vi "API_GetWindowhWnd by Window Name.vi"(8 "error in (no error)":errorcluster caption="错误输入（无错误）", 11 "窗口名称 (\"\")":string) -> (0 "error out":errorcluster caption="错误输出", 3 "窗口句柄(0)":i32)   [LabVIEW 2012, in "API.lvlib"]
uses:
  API.lvlib
  user32.dll
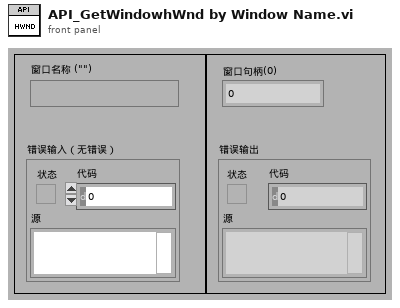
[diagram p1: front panel]
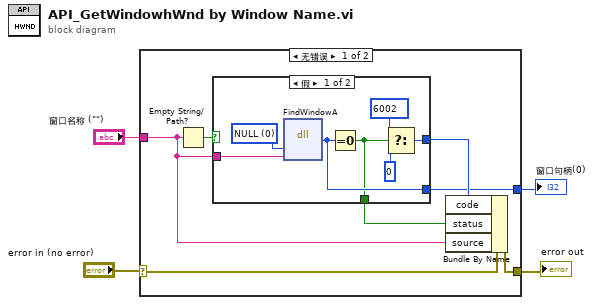
[diagram p0: block diagram]
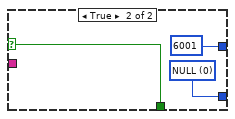
[diagram p2: hidden frame]
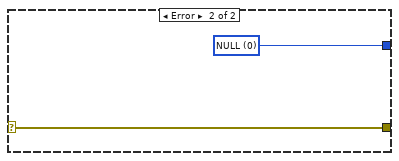
[diagram p3: hidden frame]
diagram:
  n1 = case shown="无错误" "error in (no error)" {
    selector: "error in (no error)" -> [w6 w22]
    tunnel: [w9 w22] -> w1
    tunnel: [w8 w23] -> w4
    tunnel: "窗口名称 (\"\")" -> [w5 _]
    frame No Error {
      n2 = Empty String/Path?(string/path=w5) -> (empty?=w7:bool)
      n3 = case shown="假" w7 {
        selector: w7 -> [_ w19]
        tunnel: [w18 w20] -> w8
        tunnel: [w17 w19] -> w10
        tunnel: [w16 6001] -> w11
        tunnel: w5 -> [w12 _]
        frame False {
          w13 = 0 items=["NULL"]
          n4 = dll-call lib="user32.dll" fn="FindWindowA" label="FindWindow"("lpszClassName"=w13, "lpszWindowName"=w12) -> ("hWnd"=w18:i32)  [unwired: 5 in, 2 out]
          n5 = Equal To 0?(x=w18) -> (x = 0?=w17:bool)
          n6 = Select(t=6002, s=w17, f=0) -> (s? t:f=w16:i32)
        }
        frame True {
          w20 = 0 items=["NULL"]
        }
      }
      n7 = Bundle By Name(cluster=w6, "code"=w11, "status"=w10, "source"=w5) -> (w9:errorcluster)
    }
    frame Error {
      w23 = 0 items=["NULL"]
    }
  }
  "窗口句柄(0)" <- w4
  "error out" <- w1
